vi "e.gate HighSpeedPort Get File - Read FileData.vi"(7 "Timeout (ms) [1000]":i32=1000, 8 "error in (no error)":errorcluster, 9 "Destination Path":string, 10 "File or relative Path":string, 11 "Configuration in":T1) -> (0 "error out":errorcluster, 1 "Path Out":string, 2 "data out (string)":string, 3 "Configuration out":T1)   [LabVIEW 2016]
uses:
  e.gate Configuration.ctl
  e.gate Channel Data.ctl
  e.gate Data Type.ctl
  e.gate Protocol Type.ctl
  e.gate Module  Data.ctl
  e.gateHSP_DLLhandle.ctl
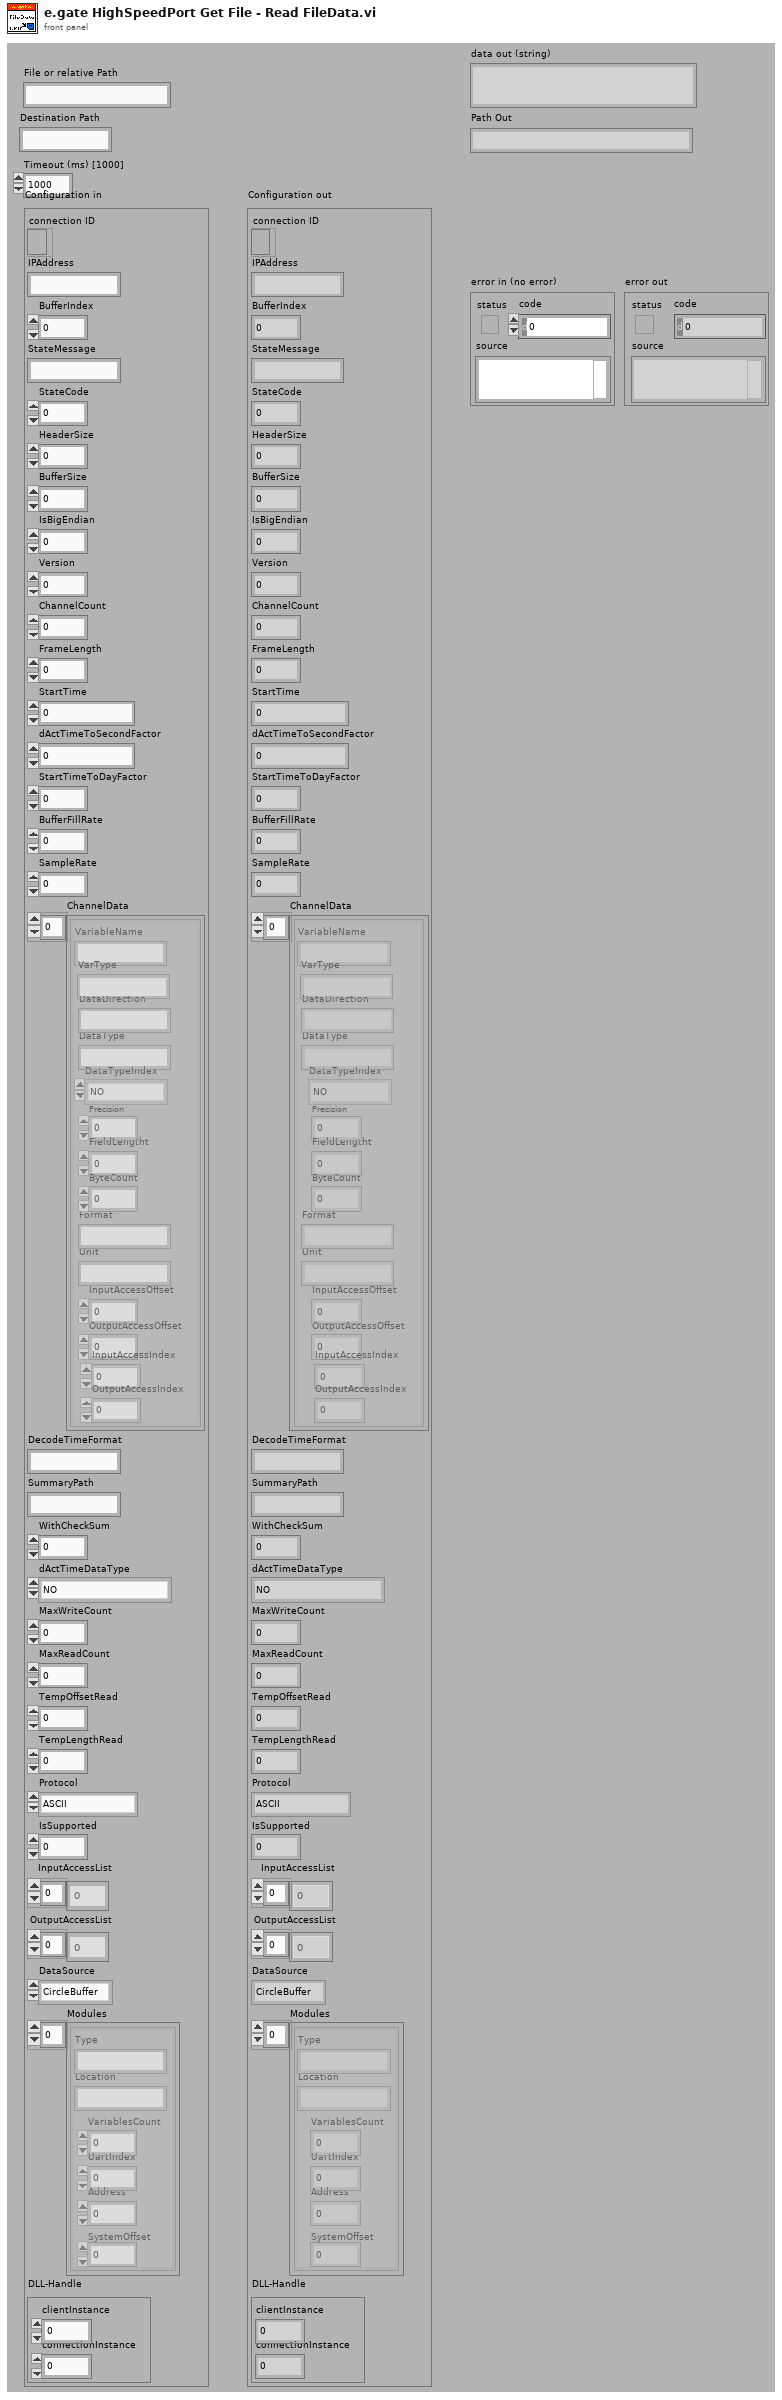
[diagram p1: front panel]
types:
  T1 = typedef "e.gate Configuration.ctl" = cluster{"connection ID":refnum<k5>, "IPAddress":string, "BufferIndex":i32, "StateMessage":string, "StateCode":i8, "HeaderSize":i32, "BufferSize":i32, "IsBigEndian":i32, "Version":i32, "ChannelCount":i32, "FrameLength":i32, "StartTime":dbl, "dActTimeToSecondFactor":dbl, "StartTimeToDayFactor":dbl, "BufferFillRate":dbl, "SampleRate":dbl, "ChannelData":T2[], "DecodeTimeFormat":string, "SummaryPath":string, "WithCheckSum":i32, "dActTimeDataType":T3, "MaxWriteCount":i32, "MaxReadCount":i32, "TempOffsetRead":i32, "TempLengthRead":i32, "Protocol":T4, "IsSupported":i32, "InputAccessList":i32[], "OutputAccessList":i32[], "DataSource":enum16{"CircleBuffer", "test.con Logger", "test.con Archive"}, "Modules":T5[], "DLL-Handle":T6}
  T2 = typedef "e.gate Channel Data.ctl" = cluster{"VariableName":string, "DataDirection":string, "DataType":string, "DataTypeIndex":T3, "Precision":i16, "FieldLengtht":i16, "ByteCount":i32, "Format":string, "Unit":string, "InputAccessOffset":i32, "OutputAccessOffset":i16, "InputAccessIndex":i16, "OutputAccessIndex":i16, "VarType":string}
  T3 = typedef "e.gate Data Type.ctl" = enum16{"NO", "BOOL", "SINT8", "USINT8", "SINT16", "USINT16", "SINT32", "USINT32", "FLOAT", "SET8", "SET16", "SET32", "DOUBLE", "SINT64", "USINT64", "SET64"}
  T4 = typedef "e.gate Protocol Type.ctl" = enum16{"ASCII", "HighspeedPort Online", "HighspeedPort Buffer", "eGateHighspeedPortDLL "}
  T5 = typedef "e.gate Module  Data.ctl" = cluster{"Type":string, "Location":string, "VariablesCount":i16, "UartIndex":i16, "Address":i16, "SystemOffset":i16}
  T6 = typedef "e.gateHSP_DLLhandle.ctl" = cluster{"clientInstance":i32, "connectionInstance":i32}
  T7 = enum16{"open", "replace", "create", "open or create", "replace or create", "replace or create with confirmation"}
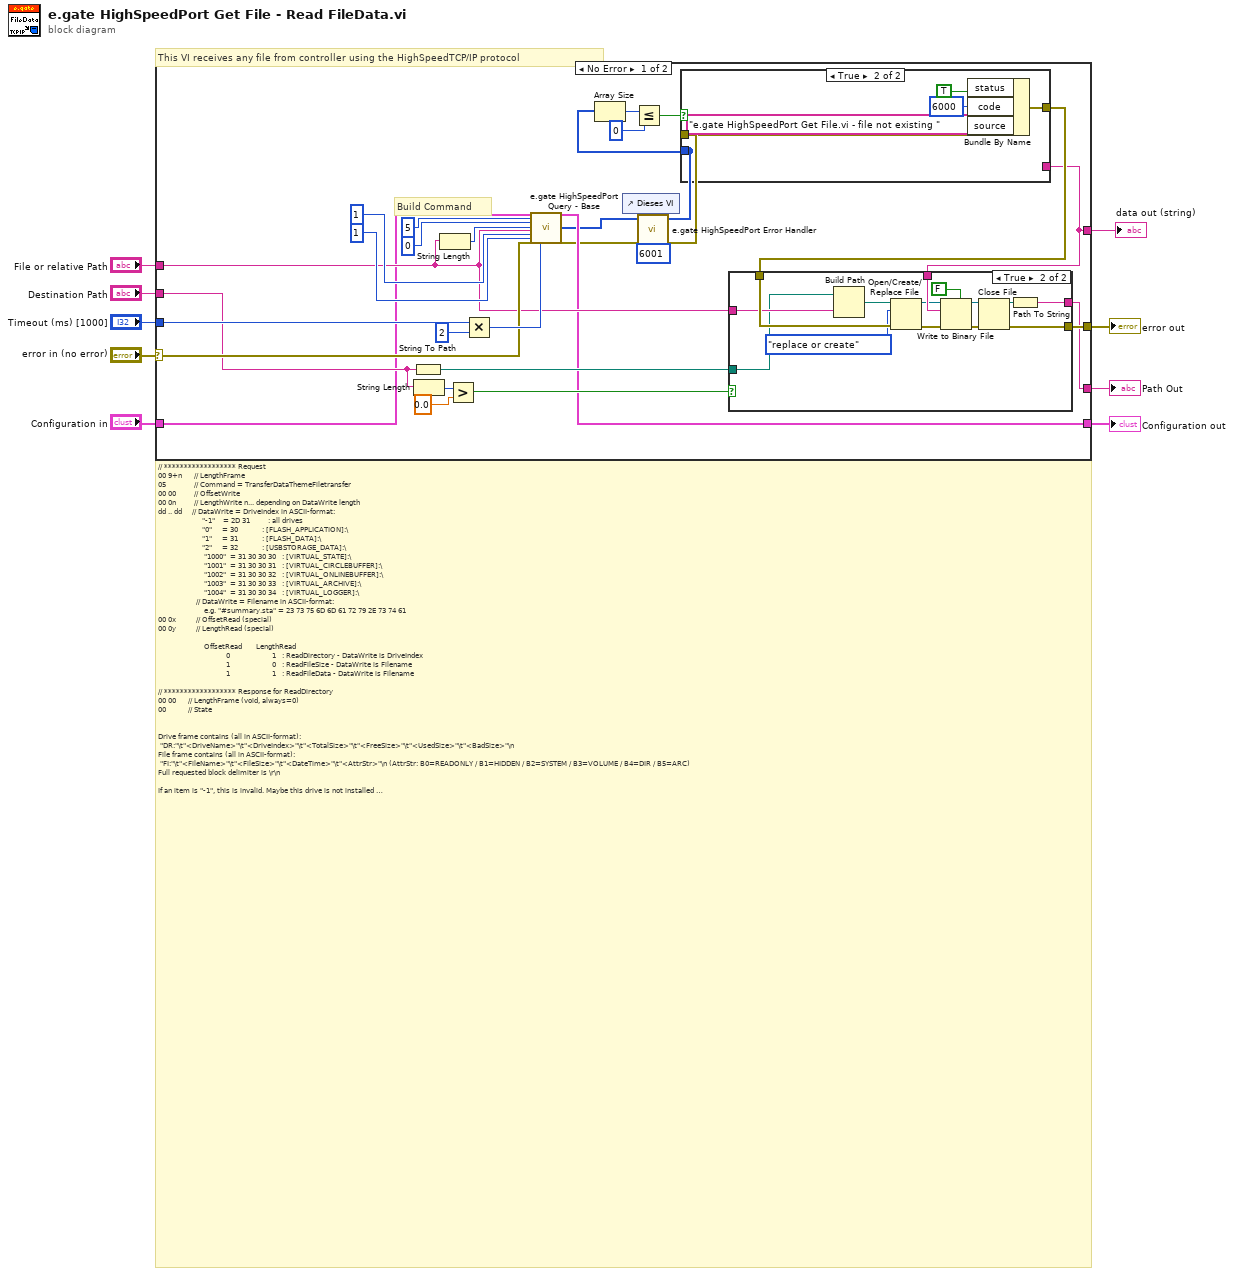
[diagram p0: block diagram]
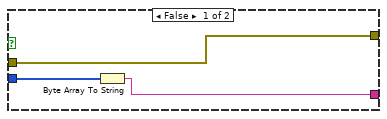
[diagram p2: hidden frame]
diagram:
  # "// ****************** Request\n00 9+n\t\t\t\t\t\t// LengthFrame\n05\t\t\t\t\t\t\t       // Command = TransferDataThemeFiletransfer\n00 00\t\t\t\t   \t\t// OffsetWrite\n00 0n\t\t\t\t\t   \t// LengthWrite n... depending on DataWrite length\ndd .. dd\t\t\t\t\t// DataWrite = DriveIndex in ASCII-format:\n\t\t\t\t\t\t\t              \t\"-1\"    = 2D 31         : all drives\n\t\t\t\t\t\t              \t\t\"0\"     = 30            : [FLASH_APPLICATION]:\\\n\t\t\t\t\t\t\t              \t\"1\"     = 31            : [FLASH_DATA]:\\\n\t\t\t              \t\t\t\t\t\"2\"     = 32            : [USBSTORAGE_DATA]:\\\n\t\t\t\t\t\t               \t\t\"1000\"  = 31 30 30 30   : [VIRTUAL_STATE]:\\\n\t\t\t\t\t\t\t               \t\"1001\"  = 31 30 30 31   : [VIRTUAL_CIRCLEBUFFER]:\\\n\t\t\t\t\t\t\t               \t\"1002\"  = 31 30 30 32   : [VIRTUAL_ONLINEBUFFER]:\\\n\t\t\t\t\t\t               \t\t\"1003\"  = 31 30 30 33   : [VIRTUAL_ARCHIVE]:\\\n\t\t\t\t\t\t               \t\t\"1004\"  = 31 30 30 34   : [VIRTUAL_LOGGER]:\\\n\t\t\t\t\t\t            \t// DataWrite = Filename in ASCII-format:\n\t\t\t\t\t\t\t               \te.g. \"#summary.sta\" = 23 73 75 6D 6D 61 72 79 2E 73 74 61\n00 0x\t\t\t\t\t\t    // OffsetRead (special)\n00 0y\t\t\t\t\t\t    // LengthRead (special)\n\n\t\t\t\t\t\t\t\t               OffsetRead      \tLengthRead\n\t\t\t\t\t\t\t                          \t0\t                  \t\t1\t\t\t: ReadDirectory - DataWrite is DriveIndex\n\t\t\t\t\t\t\t                          \t1\t\t                  \t0\t\t\t: ReadFileSize - DataWrite is Filename\n\t\t\t\t\t\t\t                          \t1\t\t\t                  1\t\t\t: ReadFileData - DataWrite is Filename\n\n// ****************** Response for ReadDirectory\n00 00\t\t\t\t\t\t// LengthFrame (void, always=0)\n00\t\t\t\t\t    \t\t// State\n\n\nDrive frame contains (all in ASCII-format):\n\t\"DR:\"\\t\"<DriveName>\"\\t\"<DriveIndex>\"\\t\"<TotalSize>\"\\t\"<FreeSize>\"\\t\"<UsedSize>\"\\t\"<BadSize>\"\\n\nFile frame contains (all in ASCII-format):\n\t\"FI:\"\\t\"<FileName>\"\\t\"<FileSize>\"\\t\"<DateTime>\"\\t\"<AttrStr>\"\\n\t(AttrStr: B0=READONLY / B1=HIDDEN / B2=SYSTEM / B3=VOLUME / B4=DIR / B5=ARC)\nFull requested block delimiter is \\r\\n\n\nIf an item is \"-1\", this is invalid. Maybe this drive is not installed or parameter is not available there !!!\n\ne.g. ReadDirectory of DriveIndex=0:\n\\x00\\x00\\x00\nDR:\\t[FLASH_APPLICATION]:\\\\t0\\t7077888\\t4878336\\t2199552\\t0\\n\nFI:\\tecpu01.bin\\t1764336\\t2008-03-11\\t10:51:40\\t0020\\n\nFI:\\tecpu01.ini\\t495\\t1980-01-01\\t12:00:00\\t0020\\n\nFI:\\tconfig.sys\\t219\\t1980-01-01\\t12:00:00\\t0020\\n\nFI:\\tfpga.bit\\t403014\\t1980-01-01\\t12:00:00\\t0020\\n\nFI:\\tftp_lic.cnf\\t538\\t2008-02-26\\t15:43:42\\t0020\\n\nFI:\\tmaster.gcf\t10750\\t2008-02-26\\t15:43:50\\t0020\\n\nFI:\\tself.ini\\t78\\t2008-03-11 09:27:36\\t0020\\n\\r\\n\n\n// ****************** Response for ReadFileSize\n00 1+n\t\t\t\t\t\t// LengthFrame\n00\t\t\t\t\t\t       \t// State\ndd .. dd\t\t\t\t\t// DataRead: Size of file in ASCII-format with length n\n\n// ****************** Response for ReadFileData\n00 1+n\t\t\t\t\t\t// LengthFrame\n00\t\t\t\t\t\t       \t// State\ndd .. dd\t\t\t\t\t// DataRead: Content of file with length n\n\n\nATTENTION: If LengthFrame is 0xFFFF, an ExtendedLengthFrame element with 4 bytes is inserted after LF LF, to make possible,\n\tto transfer more than 65534 bytes of data !!!"
  # "This VI receives any file from controller using the HighSpeedTCP/IP protocol"
  n1 = case shown="No Error" "error in (no error)" {
    selector: "error in (no error)" -> [w31 w63]
    tunnel: [w21 w64] -> w7
    tunnel: "Configuration in" -> [w22 w64]
    tunnel: [w39 w63] -> w4
    tunnel: [w38 _] -> w9
    tunnel: "Timeout (ms) [1000]" -> [w37 _]
    tunnel: "File or relative Path" -> [w23 _]
    tunnel: "Destination Path" -> [w28 _]
    tunnel: [w10 _] -> w1
    frame No Error {
      # "Build Command"
      n2 = String To Path(string=w28) -> (path=w27:path)
      n3 = String Length(string=w28) -> (length=w29:i32)
      n4 = String Length(string=w23) -> (length=w32:i32)
      n5 = Greater?(x=w29, y=0.0) -> (0:w24:bool)
      n6 = Multiply(x=w37, y=2) -> (x*y=w35:i32)
      n7 = call "e.gate HighSpeedPort Query - Base.vi"("e.gate Configuration in"=w22, "Command"=5, "OffsetWrite"=0 ("Command"), "LengthWrite"=w32, "DataWrite"=w23, "OffsetRead"=1 ("Command"), "LengthRead"=1 ("Command"), "error in (no error)"=w31, "Timeout (1000)"=w35) -> ("e.gate Configuration out"=w21:T1, "Data (out binary)"=w15:u8[], "error out"=w14:errorcluster)  [unwired: 1 in, 15 out]
      n8 = control-ref of="Dieses VI"() -> (w16:refnum<vi>)
      n9 = call "e.gate HighSpeedPort Error Handler.vi"("error code start index"=6001, "VI reference"=w16, "error in (no error)"=w14, "binary data in"=w15) -> ("error out"=w13:errorcluster, "binary out"=w11:u8[])  [unwired: 6 out]
      n10 = Array Size(array=w11) -> (size(s)=w20:i32)
      n11 = Less Or Equal?(x=w20, y=0) -> (x <= y?=w18:bool)
      n12 = case shown="True" w18 {
        tunnel: w13 -> [w42 w47]
        tunnel: [w42 w46] -> w12
        tunnel: w11 -> [w41 _]
        tunnel: [w40 _] -> w10
        frame False {
          n13 = Byte Array To String(unsigned byte array=w41) -> (string=w40:string)
        }
        frame True {
          n14 = Bundle By Name(cluster=w47, "status"=TRUE, "code"=6000, "source"="e.gate HighSpeedPort Get File.vi - file not existing ") -> (w46:errorcluster)
        }
      }
      n15 = case shown="True" w24 {
        tunnel: [w48 w62] -> w39
        tunnel: [_ w61] -> w38
        tunnel: w12 -> [w48 w60]
        tunnel: w23 -> [_ w59]
        tunnel: w10 -> [_ w58]
        tunnel: w27 -> [_ w49]
        frame False {
        }
        frame True {
          n16 = Build Path(base path=w49, name or relative path=w59) -> (appended path=w53:path)
          n17 = Open/Create/Replace File(file path (use dialog)=w53, error in=w60, operation (0:open)=T7."replace or create") -> (refnum out=w50:refnum<file>, error out=w51:errorcluster)  [unwired: 4 out]
          n18 = Write to Binary File ("Datei schreiben")(file (use dialog)=w50, data=w58, error in=w51, 5:FALSE ("prepend array or string size? (T)")) -> (refnum out=w57:refnum<file>, error out=w55:errorcluster)  [unwired: 3 out]
          n19 = Close File(refnum=w57, error in=w55) -> (path=w56:path, error out=w62:errorcluster)
          n20 = Path To String(path=w56) -> (string=w61:string)
        }
      }
    }
    frame Error {
    }
  }
  "Path Out" <- w9
  "Configuration out" <- w7
  "error out" <- w4
  "data out (string)" <- w1
